vi "Dump to String.vi"(7 "Exclude Key":bool, 8 "error in (no error)":errorcluster, 10 "Key":string, 11 "FlexWorktable in":refnum<class "FlexWorktable.lvclass">) -> (0 "error out":errorcluster, 2 "Line out":string, 3 "FlexWorktable out":refnum<class "FlexWorktable.lvclass">)   [LabVIEW 2017, in "FlexWorktable.lvclass"]
uses:
  FlexWorktable.lvclass
  FlexWorktable.lvclass/FlexWorktable.ctl
  Orient3d Class/Orient3d.lvclass
  Vec3d Class/Vec3d.lvclass
  <vilib>/Utility/Data Type/NI_Data Type.lvlib
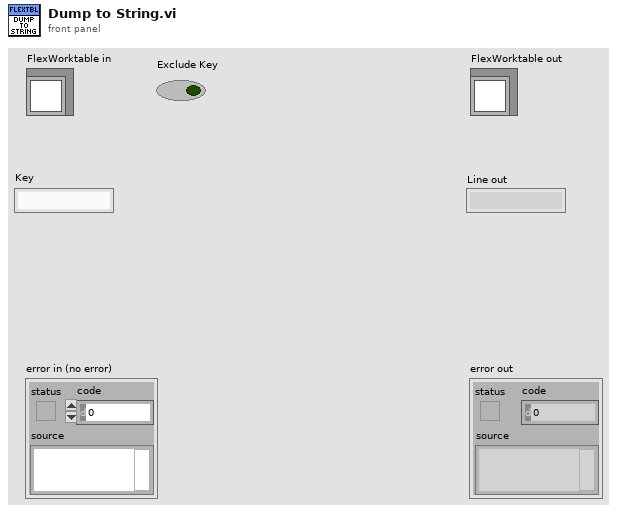
[diagram p1: front panel]
types:
  T1 = typedef "NI_Data Type.lvlib/Data Type.ctl" = enum8{"Invalid Type", "Void", "I8", "I16", "I32", "I64", "U8", "U16", "U32", "U64", "Single Float", "Double Float", "Extended Float", "Single Complex", "Double Complex", "Extended Complex", "Enum U8", "Enum U16", "Enum U32", "Enum U64", "Single Float With Unit", "Double Float With Unit", "Extended Float With Unit", "Single Complex with Unit", "Double Complex with Unit", "Extended Complex with Unit", "Boolean", "String", "Path", "Picture", "Tag", "Array", "Cluster", "Variant", "LV Variant", "Waveform", "Timestamp", "Digital Waveform", "Digital Data", "ExpressData", "Refnum", "External Data", "VI", "Poly VI", "LabVIEW Class Instance", "Fixed Point"}
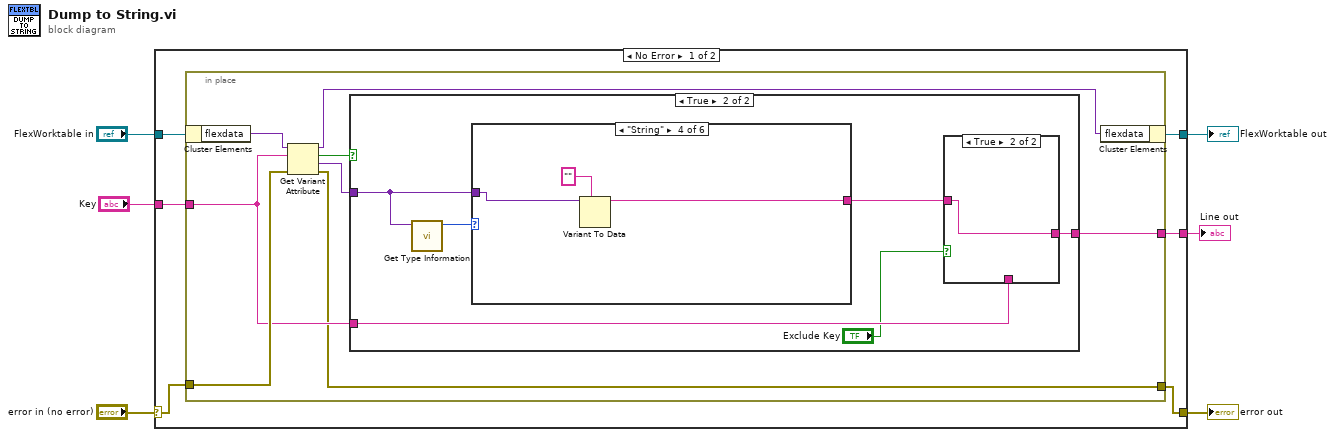
[diagram p0: block diagram]
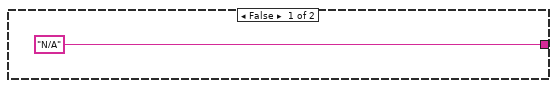
[diagram p2: hidden frame]
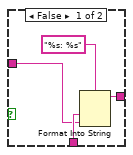
[diagram p3: hidden frame]
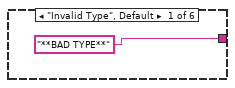
[diagram p4: hidden frame]
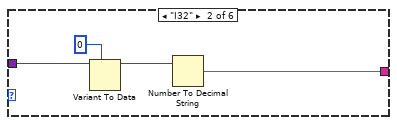
[diagram p5: hidden frame]
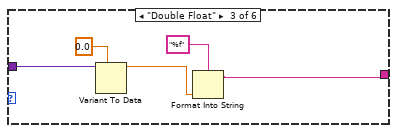
[diagram p6: hidden frame]
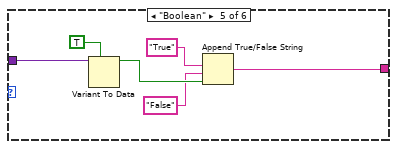
[diagram p7: hidden frame]
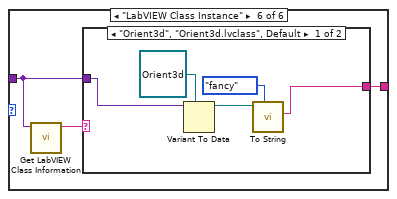
[diagram p8: hidden frame]
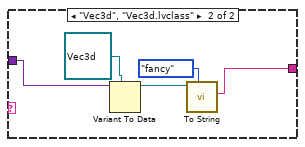
[diagram p9: hidden frame]
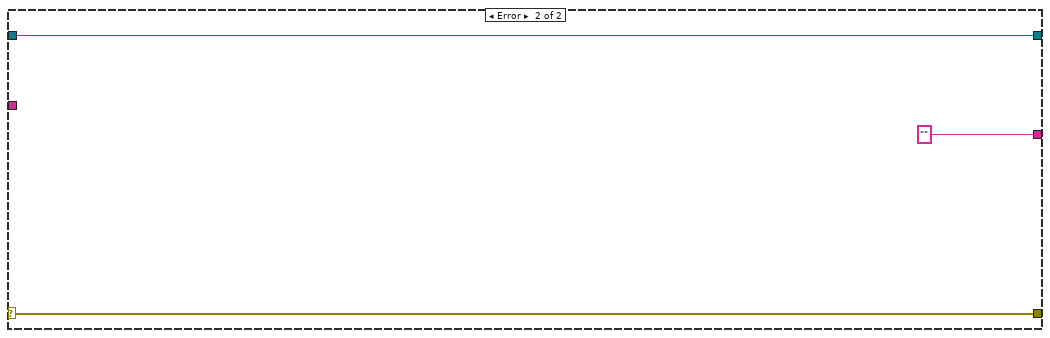
[diagram p10: hidden frame]
diagram:
  n1 = case shown="No Error" "error in (no error)" {
    selector: "error in (no error)" -> [w11 w67]
    tunnel: [w7 w67] -> w5
    tunnel: [w8 w66] -> w3
    tunnel: "FlexWorktable in" -> [w12 w66]
    tunnel: "Key" -> [w10 _]
    tunnel: [w9 ""] -> w1
    frame No Error {
      n2 = in-place {
        in-place-border: w11 -> [w19]
        in-place-border: w10 -> [w14]
        in-place-border: [w15] -> w9
        in-place-border: [w13] -> w7
        n3 = in-place-cluster #1(w12) -> ("flexdata"=w20:variant)
        n4 = Get Variant Attribute(Variant=w20, name=w14, error in=w19) -> (duplicate Variant=w17:variant, found=w18:bool, value=w16:variant, error out=w13:errorcluster)  [unwired: 1 in]
        n5 = case shown="True" w18 {
          tunnel: ["N/A" w25] -> w15
          tunnel: w16 -> [_ w27]
          tunnel: w14 -> [_ w24]
          frame False {
          }
          frame True {
            n6 = call <vilib>:"Get Type Information.vi"("Variant"=w27) -> ("Type"=w26:T1)  [unwired: 6 in, 4 out]
            n7 = case shown="\"String\"" w26 {
              tunnel: w27 -> [_ w37 w41 w44 w47 w53]
              tunnel: ["**BAD TYPE**" w34 w38 w43 w46 w52] -> w23
              frame "Invalid Type", Default {
              }
              frame "I32" {
                n8 = Variant To Data(type=0, Variant=w37) -> (data=w35:i32)  [unwired: 1 in, 1 out]
                n9 = Number To Decimal String(number=w35) -> (decimal integer string=w34:string)  [unwired: 1 in]
              }
              frame "Double Float" {
                n10 = Variant To Data(type=0.0, Variant=w41) -> (data=w39:dbl)  [unwired: 1 in, 1 out]
                n11 = Format Into String(format string="%f", w39) -> (resulting string=w38:string)  [unwired: 2 in, 1 out]
              }
              frame "String" {
                n12 = Variant To Data(type="", Variant=w44) -> (data=w43:string)  [unwired: 1 in, 1 out]
              }
              frame "Boolean" {
                n13 = Variant To Data(type=TRUE, Variant=w47) -> (data=w50:bool)  [unwired: 1 in, 1 out]
                n14 = Append True/False String(1:w50, 2:"False" ("false string"), 3:"True" ("true string")) -> (0:w46:string)  [unwired: 1 in]
              }
              frame "LabVIEW Class Instance" {
                n15 = call <vilib>:"Get LabVIEW Class Information.vi"("Variant"=w53) -> ("LabVIEW Class File Name"=w54:string)  [unwired: 8 in, 2 out]
                n16 = case shown="\"Orient3d\", \"Orient3d.lvclass\", Default" w54 {
                  tunnel: w53 -> [w57 w61]
                  tunnel: [w56 w60] -> w52
                  frame "Orient3d", "Orient3d.lvclass", Default {
                    n17 = Variant To Data(type=refnum<class "Orient3d.lvclass"> refnum ("Orient3d Class.lvclass"), Variant=w57) -> (data=w59:refnum<class "Orient3d.lvclass">)  [unwired: 1 in, 1 out]
                    n18 = call "To String.vi"("Formatting"=enum16{"plain", "fancy"}."fancy", "Orient3d in"=w59) -> ("Orient3d String"=w56:string)  [unwired: 7 in, 2 out]
                  }
                  frame "Vec3d", "Vec3d.lvclass" {
                    n19 = Variant To Data(type=refnum<class "Vec3d.lvclass"> refnum ("Vec3d Class.lvclass"), Variant=w61) -> (data=w63:refnum<class "Vec3d.lvclass">)  [unwired: 1 in, 1 out]
                    n20 = call "To String.vi"("Formatting"=enum16{"plain", "fancy"}."fancy", "Vec3d in"=w63) -> ("Vec3d String"=w60:string)  [unwired: 7 in, 2 out]
                  }
                }
              }
            }
            n21 = case shown="True" "Exclude Key" {
              tunnel: [w30 w32] -> w25
              tunnel: w24 -> [w29 _]
              tunnel: w23 -> [w28 w32]
              frame False {
                n22 = Format Into String(format string="%s: %s", w29, w28) -> (resulting string=w30:string)  [unwired: 2 in, 1 out]
              }
              frame True {
              }
            }
          }
        }
        n23 = in-place-cluster #1("flexdata"=w17) -> (w8:refnum<class "FlexWorktable.lvclass">)
      }
    }
    frame Error {
    }
  }
  "error out" <- w5
  "FlexWorktable out" <- w3
  "Line out" <- w1
